vi "Configure Preset Values.vi"(8 "error in (no error)":errorcluster, 10 "Memory Preset":dbl[][](array[numeric]) format="%.1g", 11 "VISA resource name":refnum<visa-resource-name>) -> (0 "error out":errorcluster, 3 "VISA resource name out":refnum<visa-resource-name>)   [LabVIEW 2021, in "BK Precision 169XB.lvlib"]
doc: "Returns the actual voltage level and actual current level for a desired channel."
uses:
  BK Precision 169XB.lvlib
panel:
  # "Voltage"
  # "Current"
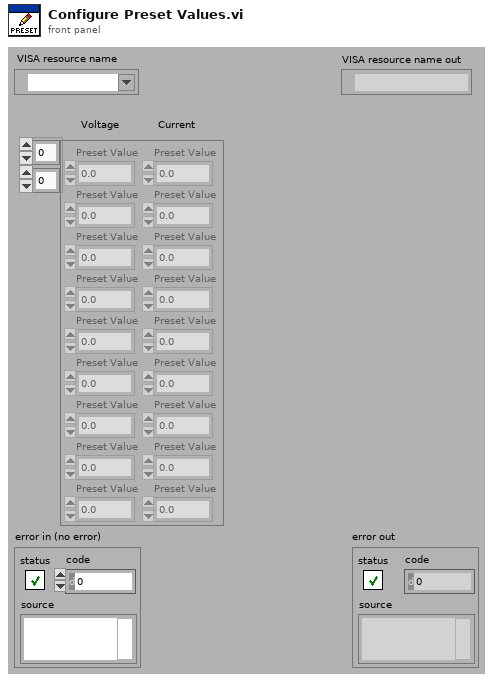
[diagram p1: front panel]
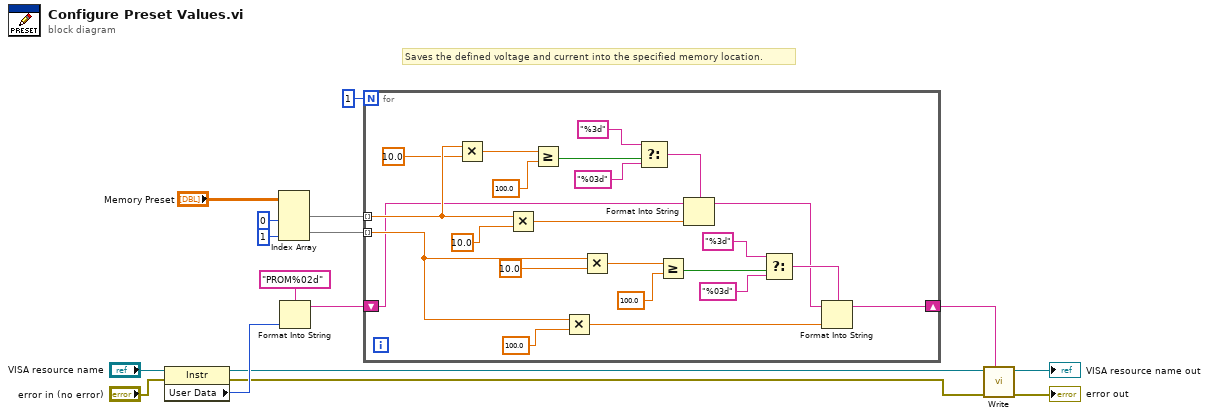
[diagram p0: block diagram]
diagram:
  # "Saves the defined voltage and current into the specified memory location."
  n1 = property class="Instr"(reference="VISA resource name", error in="error in (no error)") -> (reference out=w4:refnum<visa-resource-name>, error out=w3:errorcluster, "User Data"=w7:u32)
  n2 = Index Array(array="Memory Preset", index (col) #1=0 ("disabled index (col)"), index (col) #2=1 ("index (col)")) -> (element #1=w11:dbl[], element #2=w10:dbl[])  [unwired: 2 in]
  n3 = Format Into String(format string="PROM%02d", w7) -> (resulting string=w2:string)  [unwired: 2 in, 1 out]
  n4 = for {
    N: 1 -> [_]
    tunnel: w11 -> [w21] mode=indexing
    tunnel: w10 -> [w19] mode=indexing
    shift-right: [w22] -> w9
    shift-left: w2 -> [w17]
    n5 = Multiply(x=w21, y=10.0) -> (x*y=w38:dbl)
    n6 = Multiply(x=w21, y=10.0) -> (x*y=w32:dbl)
    n7 = Greater Or Equal?(x=w38, y=100.0) -> (x >= y?=w36:bool)
    n8 = Multiply(x=w19, y=100.0) -> (x*y=w31:dbl)
    n9 = Multiply(x=w19, y=10.0) -> (x*y=w25:dbl)
    n10 = Select(t="%3d" ("format string"), s=w36, f="%03d" ("format string")) -> (s? t:f=w33:string)
    n11 = Greater Or Equal?(x=w25, y=100.0) -> (x >= y?=w27:bool)
    n12 = Format Into String(format string=w33, initial string=w17, w32) -> (resulting string=w23:string)  [unwired: 1 in, 1 out]
    n13 = Select(t="%3d" ("format string"), s=w27, f="%03d" ("format string")) -> (s? t:f=w30:string)
    n14 = Format Into String(format string=w30, initial string=w23, w31) -> (resulting string=w22:string)  [unwired: 1 in, 1 out]
  }
  n15 = call "Write.vi"("Input String"=w9, "error in (no error)"=w3, "VISA resource name"=w4) -> ("error out"=→"error out":errorcluster, "VISA resource name out"=→"VISA resource name out":refnum<visa-resource-name>)  [unwired: 6 in, 1 out]
